vi "PropagateBeam.vi"(1 "q in":T1, 2 "Matrix":string[][](array[string])) -> (0 "q out":T1)   [LabVIEW 2011]
uses:
  <vilib>/imath/engines/lvmath/Plug In/_Char/NIMS_CH_character datatype.ctl
  <vilib>/imath/engines/lvmath/Plug In/_Char/NIMS_CH_String to Character Array.vi
  <vilib>/imath/engines/lvmath/Plug In/_Char/NIMS_CH_Character RV to String.vi
  <vilib>/imath/engines/lvmath2/RunTimeEngine/NodeEndStatement/NIMS_NodeEndStatement_Output.vi
  <instcachedir>/0/NIMS_NodeEndStatement_Output_53EC0D466D134D7ABD903AC30B43404B.lvgen/NIMS_NodeEndStatement_Output_53EC0D466D134D7ABD903AC30B43404B_007.vi
  <vilib>/imath/engines/lvmath2/RunTimeEngine/ErrorHandling/NIMS_Finalize Error.vi
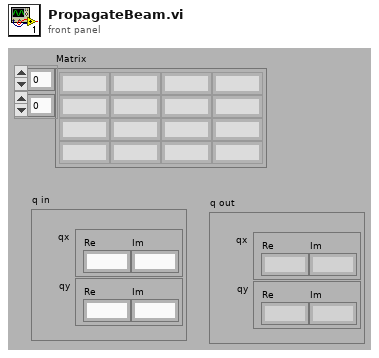
[diagram p1: front panel]
types:
  T1 = cluster{"qx":cluster{"Re":string, "Im":string}, "qy":cluster{"Re":string, "Im":string}}
  T2 = typedef "NIMS_CH_character datatype.ctl" = cluster{"Numeric":u8}
  T3 = cluster{"[0]":cluster{"qOutR":string, "qOutI":string}, "[1]":cluster{"qOutR":string, "qOutI":string}}
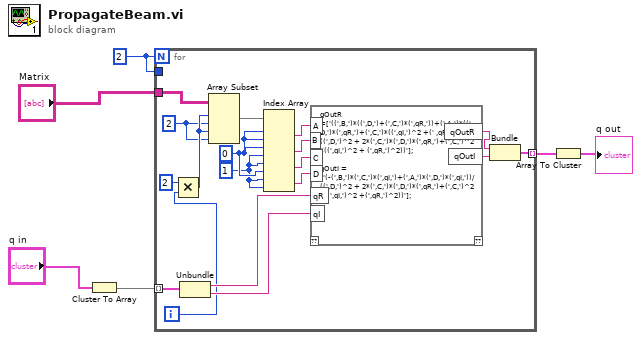
[diagram p0: block diagram]
diagram:
  w1 = 2
  n1 = Cluster To Array(cluster="q in") -> (array=w5:cluster{"Re":string, "Im":string}[])
  n2 = for {
    N: w1 -> [_]
    tunnel: w5 -> [w20] mode=indexing
    tunnel: "Matrix" -> [w24]
    tunnel: [w17] -> w3 mode=indexing
    tunnel: w1 -> [_]
    i -> [w14]
    w11 = 1 ("dimension size")
    w12 = 0 ("dimension size")
    w21 = 2 ("length")
    n3 = Multiply(x=2, y=w14) -> (x*y=w22:i32)
    n4 = Unbundle(w20) -> ("Re"=w19:string, "Im"=w18:string)
    n5 = Array Subset(array=w24, index (row)=w22, length (row)=w21, index (col)=w22, length (col)=w21) -> (w13:string[][])
    n6 = Index Array(array=w13, index (row) #1=w12, index (col) #1=w12, index (row) #2=w12, index (col) #2=w11, index (row) #3=w11, index (col) #3=w12, index (row) #4=w11, index (col) #4=w11) -> (element #1=w10:string, element #2=w9:string, element #3=w8:string, element #4=w7:string)
    n7 = mathscript code="qOutR =['((',B,')*((',D,')+(',C,')*(',qR,'))+(',A,')*((',D,')*(',qR,')+(',C,')*((',qI,')^2 +(' ,qR,')^2)))/((',D,')^2 + 2*(',C,')*(',D,')*(',qR,')+(',C,')^2 *((',qI,')^2 + (',qR,')^2))'];\n\nqOutI = ['(-(',B,')*(',C,')*(',qI,')+(',A,')*(',D,')*(',qI,'))/((',D,')^2 + 2*(',C,')*(',D,')*(',qR,')+(',C,')^2 *((',qI,')^2 +(',qR,')^2))'];"("qR"=w19, "qI"=w18, "A"=w10, "B"=w9, "C"=w8, "D"=w7) -> ("qOutR"=w16:string, "qOutI"=w15:string)  [unwired: 1 in, 1 out]
    n8 = Bundle("qOutR"=w16, "qOutI"=w15) -> (w17:cluster{"qOutR":string, "qOutI":string})  [unwired: 1 in]
  }
  n9 = Array To Cluster(array=w3) -> (cluster=→"q out":T3)
